vi "Link Control References.vi"(8 "error in (no error)":errorcluster, 10 "Control References":T1[](array[typedef]), 11 "Engine in":refnum<class "Engine.lvclass">) -> (0 "error out":errorcluster, 3 "Engine out":refnum<class "Engine.lvclass">)   [LabVIEW 2023, in "Engine.lvlib" / "Engine.lvclass"]
doc: "<b> Link Control References </b>\n<b> Engine Level </b>\nThis is the base abstraction layer. The purpose of this method is to link the control references to the class private data."
uses:
  Library/Engine.lvclass
  Custom Controls/Control Reference.ctl
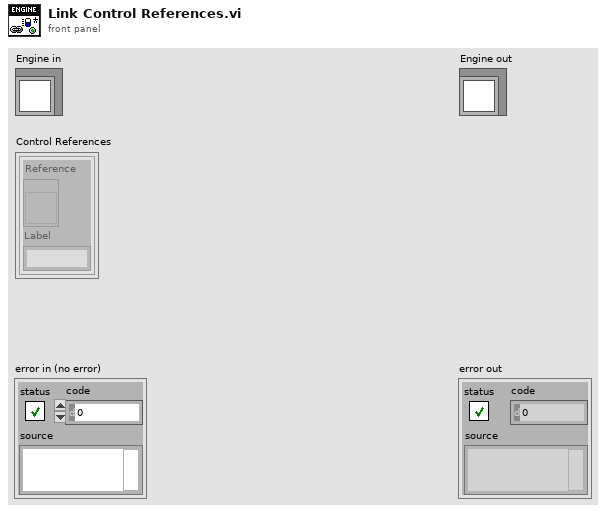
[diagram p1: front panel]
types:
  T1 = typedef "Engine.lvlib/Engine.lvclass/Control Reference.ctl" = cluster{"Reference":refnum<vi>, "Label":string}
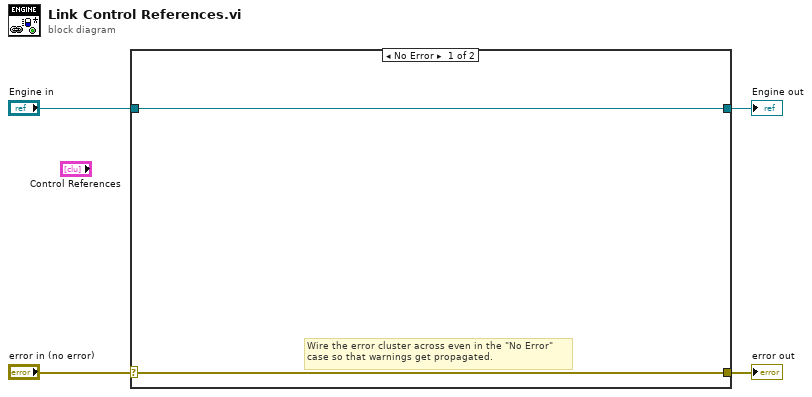
[diagram p0: block diagram]
diagram:
  n1 = case shown="No Error" "error in (no error)" {
    selector: "error in (no error)" -> [w5 w8]
    tunnel: [w5 w8] -> w3
    tunnel: [w6 w7] -> w1
    tunnel: "Engine in" -> [w6 w7]
    frame No Error {
      # "Wire the error cluster across even in the \"No Error\"\ncase so that warnings get propagated."
    }
    frame Error {
    }
  }
  "error out" <- w3
  "Engine out" <- w1
